vi "Launch Actors.vi"() -> ()   [LabVIEW 2020]
uses:
  Forms Server/Form Server/Form Server.lvclass
  C:/Program Files (x86)/National Instruments/LabVIEW 2020/vi.lib/ActorFramework/Actor/Actor.lvclass
  User Forms/TRExpRaw/TRExperimentsRaw.lvclass
  C:/Users/User/Desktop/Raman Program/Database OOP/source/Forms AF/Forms Controller/Form Window/Form Window.lvclass
  Database OOP/Database Libraries/ADODB/ADODB Class/ADODB.lvclass
  C:/Users/User/Desktop/Raman Program/Database OOP/source/Database OOP/Database Libraries/Database Interfaces/Database Advanced Schema Class/Database Adv Schema.lvclass
  User Forms/DataSets/DataSets Folder/DataSets.lvclass
  User Forms/Sample Chemical Formula/Sample Chemical Formula.lvclass
  User Forms/Samples/Samples.lvclass
  User Forms/Solutions/Solutions.lvclass
  User Forms/Users/Users/Users.lvclass
  User Forms/WorkingRange/Working Range.lvclass
  <vilib>/Utility/miscctls.llb/LVStringsAndValuesArrayTypeDef_U16.ctl
  Forms Server/Form Server Configuration/Form Server Configuration.lvclass
  Forms Server/Open Close Logic Simple Table/Open Close Logic Simple Table.lvclass
  C:/Users/User/Desktop/Raman Program/Database OOP/source/Forms AF/Forms Server/Autoclose manager/Open Close Logic.lvclass
  Forms Server/Autoclose manager/Form ID.ctl
  Database OOP/Database Libraries/ADODB/UDL Connection Class/UDL Connection.lvclass
  C:/Users/User/Desktop/Raman Program/Database OOP/source/Database OOP/Database Libraries/Database Interfaces/Database Connection Class/Database Connection.lvclass
  Forms Model/Form Model Configuration/Form Model Configuration Class/Form Model Configuration.lvclass
  Forms Server/Form Server Configuration/Form Server Configuration.lvclass/Form Server Configuration.ctl
  Forms Server/Form Server/Form Server.lvclass/Form Server.ctl
  Forms Server/Form Server Messages Messages/Open Form Msg/Open Form Msg.lvclass/Open Form Msg.ctl
  <vilib>/ActorFramework/Message Enqueuer/Message Enqueuer.lvclass/Message Enqueuer.ctl
  Forms Server/Form Server Messages Messages/Get Table Object Msg/Get Table Object Msg.lvclass/Get Table Object Msg.ctl
  <vilib>/ActorFramework/Reply Msg/Reply Msg.lvclass/Reply Msg.ctl
  Forms Server/Form Server Messages Messages/Update Form Msg/Update Form Msg.lvclass/Update Form Msg.ctl
  <vilib>/ActorFramework/Message Enqueuer/Enqueue.vi
  <vilib>/ActorFramework/Reply Msg/Send Message And Wait For Response.vi
  <vilib>/MGI/Panel Manager/Panel/Panel/Subpanel/Subpanel.lvclass
  C:/Program Files (x86)/National Instruments/LabVIEW 2020/vi.lib/MGI/Panel Manager/Panel/Panel/Panel.lvclass
  <vilib>/MGI/Panel Manager/Panel/Panel/Window/Window.lvclass
  Forms Model/Model Panel Logic/Model Panel Logic Nested Window.lvclass
  C:/Users/User/Desktop/Raman Program/Database OOP/source/Forms AF/Forms Model/Form Model Interfaces/Model Panel Logic Interface/Model Panel Logic.lvclass
  Database OOP/Table Libraries/Basic Table/Configuration/Table Configuration Adv Schema DB/Table Configuration Adv Schema DB.lvclass
  C:/Users/User/Desktop/Raman Program/Database OOP/source/Database OOP/Table Libraries/Table Configuration Interface/Table Configuration Interface.lvclass
  Forms Controller/Configuration/Form from Table Configuration/Form from Table Configuration.lvclass
  C:/Users/User/Desktop/Raman Program/Database OOP/source/Forms AF/Forms Controller/Configuration/Controller Configuration/Panel Form Controller Configuration.lvclass
  Forms Controller/Form Window/Form Window.lvclass
  C:/Users/User/Desktop/Raman Program/Database OOP/source/Forms AF/Forms Controller/Form Controller/Panel Form Controller.lvclass
  Forms Server/Form Server Messages Messages/Open Form Msg/Open Form Msg.lvclass
  C:/Program Files (x86)/National Instruments/LabVIEW 2020/vi.lib/ActorFramework/Message/Message.lvclass
  Forms Server/Form Server Messages Messages/Get Table Object Msg/Get Table Object Msg.lvclass
  C:/Program Files (x86)/National Instruments/LabVIEW 2020/vi.lib/ActorFramework/Reply Msg/Reply Msg.lvclass
  <vilib>/ActorFramework/Reply Msg/Reply Msg.lvclass
  Forms Server/Form Server Messages Messages/Update Form Msg/Update Form Msg.lvclass
  <vilib>/ActorFramework/Stop Msg/Stop Msg.lvclass
  Database OOP/Table Libraries/Basic Table/Configuration/Table Configuration Adv Schema DB/Table Constructor Adv Schema DB.vi
  Forms Controller/Configuration/Form from Table Configuration/Constructor by Table Config.vi
  <vilib>/MGI/Panel Manager/Panel/Panel/Window/Window.vi
  <vilib>/MGI/Panel Manager/Panel/Panel/Subpanel/Subpanel.vi
  <vilib>/ActorFramework/Message Priority Queue/Priority Enqueue.vi
  Database OOP/Table Libraries/Basic Table/Basic Table Class/Basic Table.lvclass
  <vilib>/ActorFramework/Actor/Actor.lvclass
  <vilib>/MGI/Panel Manager/Panel/Panel.lvlib
  Forms Server/Form Server Interfaces.lvlib
  Forms Controller/Panel Form Controller.lvlib
  Database OOP/Table Libraries/Table.lvlib
  C:/Users/User/Desktop/Raman Program/Database OOP/source/Database OOP/Database Libraries/Database Interfaces/Database Interface Class/Database Interface.lvclass
  C:/Users/User/Desktop/Raman Program/Database OOP/source/Database OOP/Database Libraries/ADODB/ADODB Class/ADODB.lvclass
  C:/Users/User/Desktop/Raman Program/Database OOP/source/Database OOP/Table Libraries/Basic Table/Configuration/Table Configuration Class/Table Configuration.lvclass
  C:/Users/User/Desktop/Raman Program/Database OOP/source/Database OOP/Table Libraries/Basic Table/Configuration/Table Configuration Adv Schema DB/Table Configuration Adv Schema DB.lvclass
panel:
  out "Table Control":string[][](table)
  in  "Form Selector":u16(ring) items=["Forms.lvlib:TRExperimentsRaw.lvclass", "Forms.lvlib:DataSets.lvclass", "Forms.lvlib:Sample Chemical Formula.lvclass", "Forms.lvlib:Samples.lvclass", "Forms.lvlib:Solutions.lvclass", "Forms.lvlib:Users.lvclass", "Forms.lvlib:Working Range.lvclass"]
  in  "stop":bool
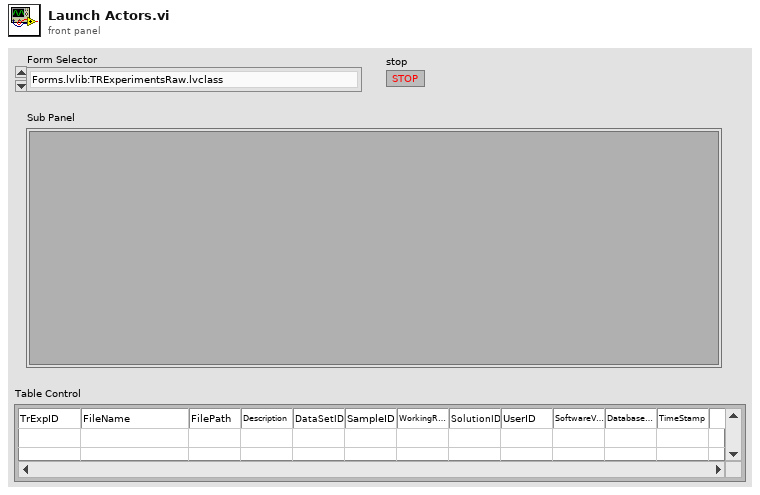
[diagram p1: front panel]
types:
  T1 = typedef "Form Server Interfaces.lvlib/Form ID.ctl" = cluster{"Name":string, "Panel type":string}
  T2 = typedef "LVStringsAndValuesArrayTypeDef_U16.ctl" = cluster{"String":string, "Value":u16}[]
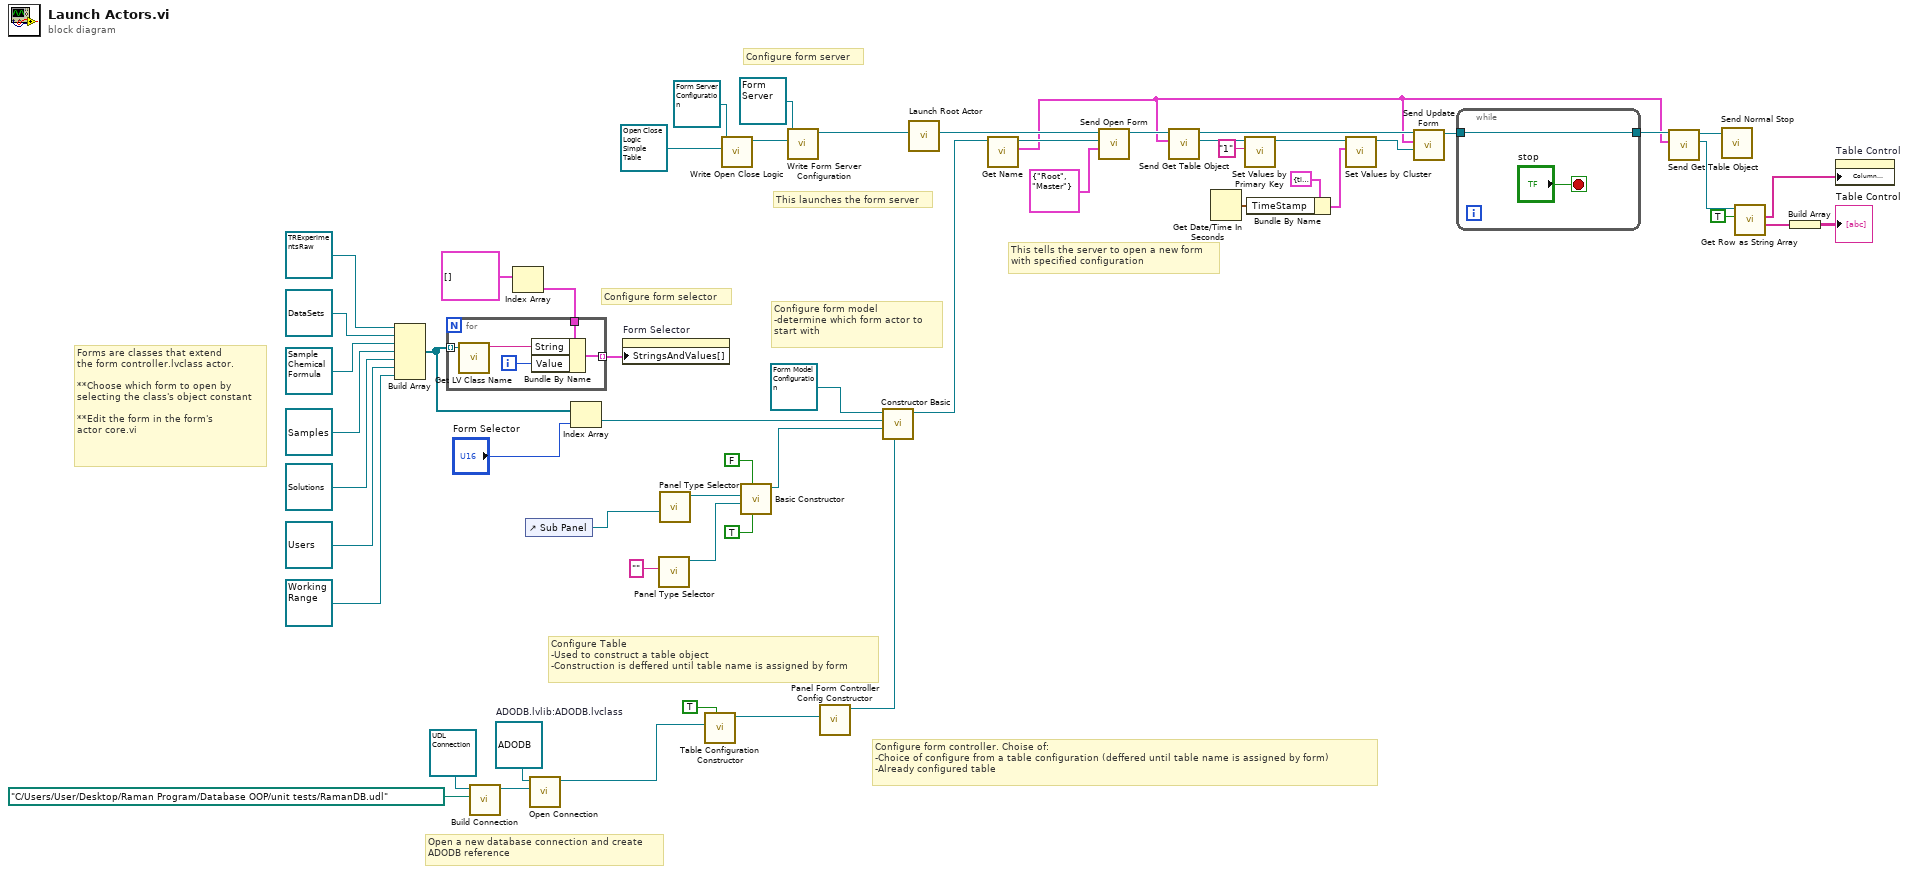
[diagram p0: block diagram]
diagram:
  w56 = refnum<class "ADODB.lvclass"> refnum  # ADODB.lvlib:ADODB.lvclass
  # "This tells the server to open a new form\nwith specified configuration"
  # "This launches the form server"
  # "Configure form controller. Choise of:\n-Choice of configure from a table configuration (deffered until table name is assigned by form)\n-Already configured table"
  # "Configure Table\n-Used to construct a table object\n-Construction is deffered until table name is assigned by form"
  # "Forms are classes that extend\nthe form controller.lvclass actor.\n\n**Choose which form to open by\nselecting the class's object constant\n\n**Edit the form in the form's\nactor core.vi"
  # "Open a new database connection and create\nADODB reference"
  # "Configure form model\n-determine which form actor to\nstart with"
  # "Configure form selector"
  # "Configure form server"
  n1 = Build Array(refnum<class "TRExperimentsRaw.lvclass"> refnum ("Forms.lvlib:TRExperimentsRaw.lvclass"), refnum<class "DataSets.lvclass"> refnum ("Forms.lvlib:DataSets.lvclass"), refnum<class "Sample Chemical Formula.lvclass"> refnum ("Forms.lvlib:Sample Chemical Formula.lvclass"), refnum<class "Samples.lvclass"> refnum ("Forms.lvlib:Samples.lvclass"), refnum<class "Solutions.lvclass"> refnum ("Forms.lvlib:Solutions.lvclass"), refnum<class "Users.lvclass"> refnum ("Forms.lvlib:Users.lvclass"), refnum<class "Working Range.lvclass"> refnum ("Forms.lvlib:Working Range.lvclass")) -> (w45:refnum<class "Form Window.lvclass">[])
  n2 = call "Build Connection.vi"("*.udl file path"=path "C:/Users/User/Desktop/Raman Program/Database OOP/unit tests/RamanDB.udl", "UDL Connection in"=refnum<class "UDL Connection.lvclass"> refnum) -> ("UDL Connection out"=w36:refnum<class "UDL Connection.lvclass">)  [unwired: 8 in, 1 out]
  n3 = Index Array(array=T2 [] ("Strings And Values []")) -> (element=w47:cluster{"String":string, "Value":u16})  [unwired: 1 in]
  n4 = for {
    tunnel: w45 -> [w61] mode=indexing
    tunnel: w47 -> [w60]
    tunnel: [w57] -> w46 mode=indexing
    i -> [w58]
    n5 = call <vilib>:"Get LV Class Name.vi"("object"=w61) -> ("class name"=w59:string)  [unwired: 9 in, 1 out]
    n6 = Bundle By Name(cluster=w60, "String"=w59, "Value"=w58) -> (w57:cluster{"String":string, "Value":u16})
  }
  n7 = control-ref of="Sub Panel"() -> (w7:refnum<vi>)
  n8 = call-dynamic "Open Connection.vi"("Connection"=w36, "ADODB in"=w56) -> ("ADODB out"=w31:refnum<class "ADODB.lvclass">)  [unwired: 8 in, 1 out]
  n9 = Index Array(array=w45, index="Form Selector") -> (element=w33:refnum<class "Form Window.lvclass">)
  n10 = property on="Form Selector" class="Ring (strict)"("StringsAndValues[]"=w46) -> ()  [unwired: 2 in, 2 out]
  n11 = call-poly <vilib>:"Panel Type Selector.vi"("Default Title"="") -> ("Window out"=w4:refnum<class "Window.lvclass">)  [unwired: 9 in, 1 out]
  n12 = call-poly <vilib>:"Panel Type Selector.vi"("Sub Panel"=w7) -> ("Subpanel Out"=w5:refnum<class "Subpanel.lvclass">)  [unwired: 9 in, 1 out]
  n13 = call-poly "Table Configuration Constructor.vi"("Defer Constructor (F)"=TRUE, "Database"=w31) -> ("Table Configuration Adv Schema DB out"=w32:refnum<class "Table Configuration Adv Schema DB.lvclass">)  [unwired: 8 in, 1 out]
  n14 = call "Write Open Close Logic.vi"("Form Server Interfaces.lvlib:Open Close Logic.lvclass"=refnum<class "Open Close Logic Simple Table.lvclass"> refnum ("Open Close Logic Simple Table.lvlib:Open Close Logic Simple Table.lvclass"), "Form Server Configuration in"=refnum<class "Form Server Configuration.lvclass"> refnum ("Form Server Configuration.lvlib:Form Server Configuration.lvclass")) -> ("Form Server Configuration out"=w41:refnum<class "Form Server Configuration.lvclass">)  [unwired: 8 in, 1 out]
  n15 = call "Basic Constructor.vi"("Nested panels for additional? (T)"=TRUE, "Nested panels for root? (F)"=FALSE, "Additional Panels (window)"=w4, "Root Panel"=w5) -> ("Model Panel Logic out"=w3:refnum<class "Model Panel Logic Nested Window.lvclass">)  [unwired: 6 in, 1 out]
  n16 = call "Write Form Server Configuration.vi"("Form Server Configuration.lvlib:Form Server Configuration.lvclass"=w41, "Form Server in"=refnum<class "Form Server.lvclass"> refnum ("Form Server.lvlib:Form Server.lvclass")) -> ("Form Server out"=w42:refnum<class "Form Server.lvclass">)  [unwired: 8 in, 1 out]
  n17 = call-poly "Panel Form Controller Config Constructor.vi"("Table Configuration"=w32) -> ("Form from Table Configuration out"=w6:refnum<class "Form from Table Configuration.lvclass">)  [unwired: 9 in, 1 out]
  n18 = call "Constructor Basic.vi"("Controller Config"=w6, "Panel Logic"=w3, "Panel Form Controller"=w33, "Form Model Configuration in"=refnum<class "Form Model Configuration.lvclass"> refnum) -> ("Form Model Configuration out"=w28:refnum<class "Form Model Configuration.lvclass">)  [unwired: 6 in, 1 out]
  n19 = call <vilib>:"Launch Root Actor.vi"("Actor"=w42) -> ("Actor's Enqueuer"=w38:refnum<class "Message Enqueuer.lvclass">)  [unwired: 9 in, 1 out]
  n20 = call-dynamic "Get Name.vi"("Form Configuration in"=w28) -> ("Form ID"=w16:T1, "Form Configuration out"=w27:refnum<class "Form Model Configuration.lvclass">)  [unwired: 8 in, 1 out]
  n21 = call "Send Open Form.vi"("Caller Name"=T1 {"Name"="Root", "Panel type"="Master"}, "Form Config"=w27, "Message Enqueuer"=w38) -> ("Message Enqueuer out"=w19:refnum<class "Message Enqueuer.lvclass">)  [unwired: 7 in, 1 out]
  n22 = call "Send Get Table Object.vi"("Form ID"=w16, "Message Enqueuer"=w19) -> ("Table"=w11:refnum<class "Basic Table.lvclass">, "Message Enqueuer out"=w18:refnum<class "Message Enqueuer.lvclass">)  [unwired: 6 in, 2 out]
  n23 = Get Date/Time In Seconds() -> (seconds since 1Jan1904=w14:timestamp)
  n24 = call "Set Values by Primary Key.vi"("Primary Key Value"="1", "Table in"=w11) -> ("Table out"=w10:refnum<class "Basic Table.lvclass">)  [unwired: 8 in, 1 out]
  n25 = Bundle By Name(cluster=cluster{"TimeStamp":timestamp} {"TimeStamp"=timestamp(0 s since 1904-01-01)} ("input cluster"), "TimeStamp"=w14) -> (w13:cluster{"TimeStamp":timestamp})
  n26 = call "Set Values by Cluster.vi"("Cluster"=w13, "Table in"=w10) -> ("Table out"=w12:refnum<class "Basic Table.lvclass">)  [unwired: 8 in, 1 out]
  n27 = call "Send Update Form.vi"("Table"=w12, "Form ID"=w16, "Message Enqueuer"=w18) -> ("Message Enqueuer out"=w17:refnum<class "Message Enqueuer.lvclass">)  [unwired: 7 in, 1 out]
  n28 = while {
    tunnel: w17 -> [w63]
    tunnel: [w63] -> w21
    stop <- "stop" stop-if-true
  }
  n29 = call "Send Get Table Object.vi"("Form ID"=w16, "Message Enqueuer"=w21) -> ("Table"=w26:refnum<class "Basic Table.lvclass">, "Message Enqueuer out"=w20:refnum<class "Message Enqueuer.lvclass">)  [unwired: 6 in, 2 out]
  n30 = call <vilib>:"Send Normal Stop.vi"("Message Enqueuer"=w20) -> ()  [unwired: 10 in, 1 out]
  n31 = call "Get Row as String Array.vi"("Keep DB Column Order (F)"=TRUE, "Table in"=w26) -> ("Row Values"=w24:string[], "Column Names"=w22:string[])  [unwired: 6 in, 2 out]
  n32 = Build Array(w24) -> (→"Table Control":string[][])
  n33 = property on="Table Control" class="Tbl (strict)"("Column Headers[]"=w22) -> ()  [unwired: 2 in, 2 out]
